vi "Multiplexer UI.vi"() -> ()   [LabVIEW 2021]
panel:
  out "output":dbl
  in  "select(ch3&4)":bool
  in  "select(ch1&2)":bool
  in  "ch4":dbl
  in  "ch3":dbl
  in  "ch2":dbl
  in  "ch1":dbl
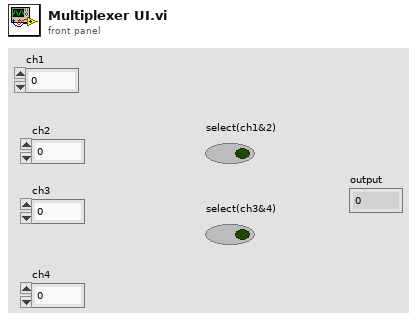
[diagram p1: front panel]
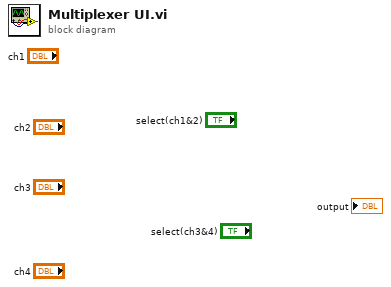
[diagram p0: block diagram]
diagram:
